vi "Create Pattern Script - Rd Collect Frame.vi"(8 "error in (no error)":errorcluster, 10 "FRM Data":T1 {"Addr" format="%x"; "Data" format="%x"}, 11 "SPI 4W Pattern Creator in":refnum<class "SPI 4W Pattern Creator.lvclass">) -> (0 "error out":errorcluster, 2 "String":string, 3 "SPI 4W Pattern Creator out":refnum<class "SPI 4W Pattern Creator.lvclass">)   [LabVIEW 2018, in "SPI 4W Pattern Creator.lvlib" / "SPI 4W Pattern Creator.lvclass"]
uses:
  SPI 4W Pattern Creator.lvclass
  Ctls/Frame Data - SPI_3W.ctl
  Ctls/RW Options.ctl
  Protocols/SPI Root Pattern Creator.lvlibp/Plugins/SouceCode/SPI_Pattern Creator/SPI Root/Data Type.ctl
  Protocols/SPI Root Pattern Creator.lvlibp/Plugins/SouceCode/SPI_Pattern Creator/SPI Root/Special Frame Type.ctl
  Protocols/SPI Root Pattern Creator.lvlibp/Plugins/SouceCode/SPI_Pattern Creator/SPI Root/SPI Root Pattern Creator.lvclass
  C:/P4 Workspace/PC Client/Solutions/5g_eap/trunk/1.0/HiSi5GmmWave/Pattern_Gen_Tool/Plugins/Protocols/SPI Root Pattern Creator.lvlibp/Plugins/SouceCode/SPI_Pattern Creator/SPI Root/SPI Root Pattern Creator.lvclass
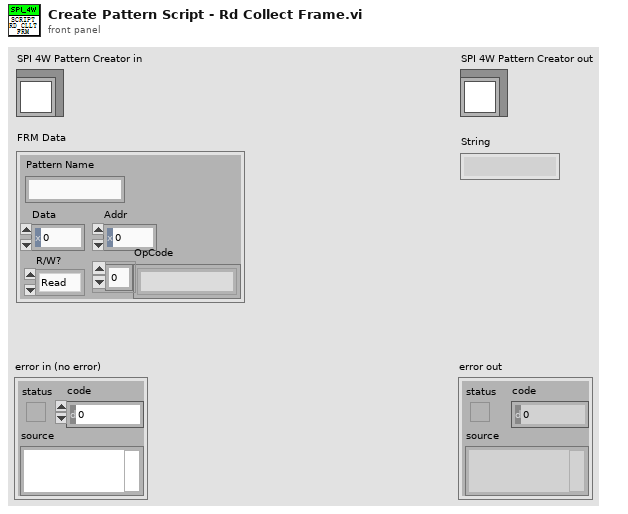
[diagram p1: front panel]
types:
  T1 = typedef "Frame Data - SPI_3W.ctl" = cluster{"Pattern Name":string, "Data":u16, "Addr":u16, "OpCode":string[], "R/W?":T2}
  T2 = typedef "RW Options.ctl" = enum16{"Read", "Write", "R/W"}
  T3 = typedef "SPI Root Pattern Creator.lvlibp/SPI Root Pattern Creator.lvclass/Special Frame Type.ctl" = enum16{"SPI 4W FRM Start", "SPI 4W Wait", "SPI 4W FRM End", "SPI 4W Write Cmd", "SPI Rd Collect Cmd", "SPI Rd Value Cmd", "SPI 3W FRM Start", "SPI 3W Write Cmd", "SPI 3W FRM End", "SPI 3W Wait", "SPI 3W Rd Cmd"}
  T4 = typedef "SPI Root Pattern Creator.lvlibp/SPI Root Pattern Creator.lvclass/Data Type.ctl" = enum16{"Drive", "Compare", "Read"}
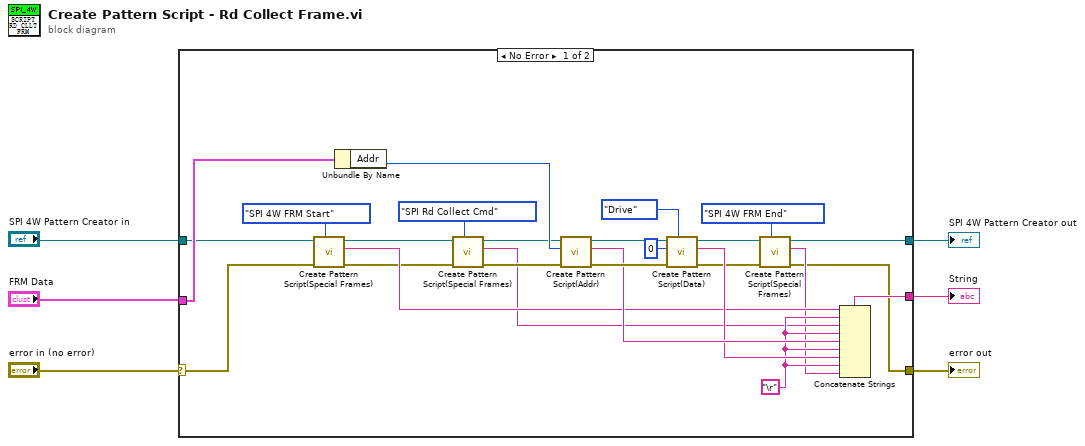
[diagram p0: block diagram]
diagram:
  n1 = case shown="No Error" "error in (no error)" {
    selector: "error in (no error)" -> [w23 w33]
    tunnel: "FRM Data" -> [w32 _]
    tunnel: "SPI 4W Pattern Creator in" -> [w21 w34]
    tunnel: [w12 w34] -> w3
    tunnel: [w10 w33] -> w2
    tunnel: [w24 _] -> w1
    frame No Error {
      w26 = "\r"
      n2 = call "Create Pattern Script(Special Frames).vi"("Special Frame Type"=Special_Frame_Type."SPI 4W FRM Start", "error in (no error)"=w23, "SPI Root Pattern Creator in"=w21) -> ("error out"=w19:errorcluster, "String out"=w22:string, "SPI Root Pattern Creator out"=w20:refnum<class "SPI 4W Pattern Creator.lvclass">)  [unwired: 6 in]
      n3 = Unbundle By Name(w32) -> ("Addr"=w29:u16)
      n4 = call "Create Pattern Script(Special Frames).vi"("Special Frame Type"=Special_Frame_Type."SPI Rd Collect Cmd", "error in (no error)"=w19, "SPI Root Pattern Creator in"=w20) -> ("error out"=w18:errorcluster, "String out"=w16:string, "SPI Root Pattern Creator out"=w17:refnum<class "SPI 4W Pattern Creator.lvclass">)  [unwired: 6 in]
      n5 = call-dynamic "Create Pattern Script(Addr).vi"("error in (no error)"=w18, "Addr"=w29, "SPI 4W Pattern Creator in"=w17) -> ("error out"=w31:errorcluster, "String"=w28:string, "SPI 4W Pattern Creator out"=w30:refnum<class "SPI 4W Pattern Creator.lvclass">)  [unwired: 6 in]
      n6 = call-dynamic "Create Pattern Script(Data).vi"("Data Type"=Data_Type."Drive", "error in (no error)"=w31, "Data"=u16 0, "SPI 4W Pattern Creator in"=w30) -> ("error out"=w13:errorcluster, "String"=w27:string, "SPI 4W Pattern Creator out"=w14:refnum<class "SPI 4W Pattern Creator.lvclass">)  [unwired: 5 in]
      n7 = call "Create Pattern Script(Special Frames).vi"("Special Frame Type"=Special_Frame_Type."SPI 4W FRM End", "error in (no error)"=w13, "SPI Root Pattern Creator in"=w14) -> ("error out"=w10:errorcluster, "String out"=w11:string, "SPI Root Pattern Creator out"=w12:refnum<class "SPI 4W Pattern Creator.lvclass">)  [unwired: 6 in]
      n8 = Concatenate Strings(w22, w26, w16, w26, w28, w26, w27, w26, w11) -> (w24:string)
    }
    frame Error {
    }
  }
  "error out" <- w2
  "SPI 4W Pattern Creator out" <- w3
  "String" <- w1
